vi "WPI_CAN_Enumerate.vi"(8 "error in (no error)":errorcluster) -> (0 "error out":errorcluster, 2 "Device Numbers":u8[](array[numeric]))   [LabVIEW 2017]
doc: "Broadcast the Enumerate command to the CAN bus and return the device numbers that respond."
uses:
  <vilib>/Rock Robotics/WPI/CAN/WPI_CAN_SystemMessageIDs.ctl
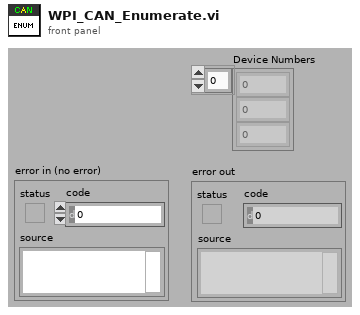
[diagram p1: front panel]
types:
  T1 = typedef "WPI_CAN_SystemMessageIDs.ctl" = u32
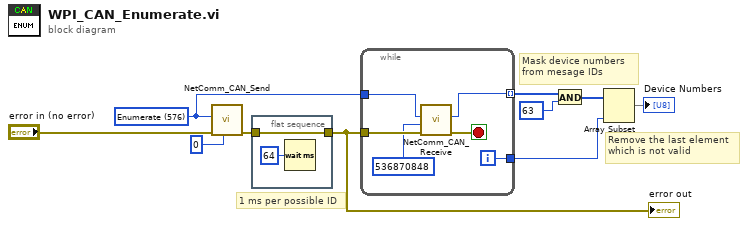
[diagram p0: block diagram]
diagram:
  w10 = T1 576 items=["Device Assignment"=128, "Device Query"=2147483840, "Sync Update"=384, "Firmware Update"=448, "Firmware Version"=2147484160, "Enumerate"=576] ("CAN System Message IDs")
  # "Remove the last element\nwhich is not valid"
  # "1 ms per possible ID"
  # "Mask device numbers\nfrom mesage IDs"
  n1 = call <vilib>:"NetComm_CAN_Send.vi"("Period (ms)"=0, "error in (no error)"="error in (no error)", "Message ID"=w10) -> ("error out"=w2:errorcluster)  [unwired: 1 in, 7 out]
  n2 = flat-sequence {
    tunnel: [w12] -> w3
    tunnel: w2 -> [w12]
    frame #0 {
      n3 = Wait (ms)(milliseconds to wait=u32 64) -> ()  [unwired: 1 out]
    }
  }
  n4 = while {
    tunnel: w3 -> [w18]
    tunnel: w10 -> [w17]
    tunnel: [w15] -> w9 mode=indexing
    tunnel: [w14] -> w6
    i -> [w14]
    stop <- w16 stop-if-true
    n5 = call <vilib>:"NetComm_CAN_Receive.vi"("error in (no error)"=w18, "Message ID Mask"=u32 536870848, "Message ID"=w17) -> ("error out"=w16:errorcluster, "Message ID Out"=w15:u32)  [unwired: 7 out]
  }
  n6 = And(x=w9, y=u8 63 ("Message ID Out")) -> (x .and. y?=w7:u32[])
  n7 = Array Subset(array=w7, length=w6) -> (→"Device Numbers":u32[])  [unwired: 1 in]
  "error out" <- w3
